vi "ProducerConsumerEvents_Queue.vi"() -> ()   [LabVIEW 2018]
doc: "Use this template to build a producer/consumer design pattern with events to produce queue items. Use this design pattern instead of the User Interface Event Handler pattern for user interfaces when you want to execute code asynchronously in response to an event without slowing the user interface responsiveness."
panel:
  in  "stop 3":bool
  in  "Enqueue Element 3":bool
  in  "stop 2":bool
  in  "Enqueue Element 2":bool
  out "data (can be any type)":string
  in  "Enqueue Element":bool
  in  "stop":bool
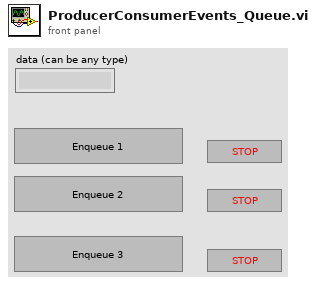
[diagram p1: front panel]
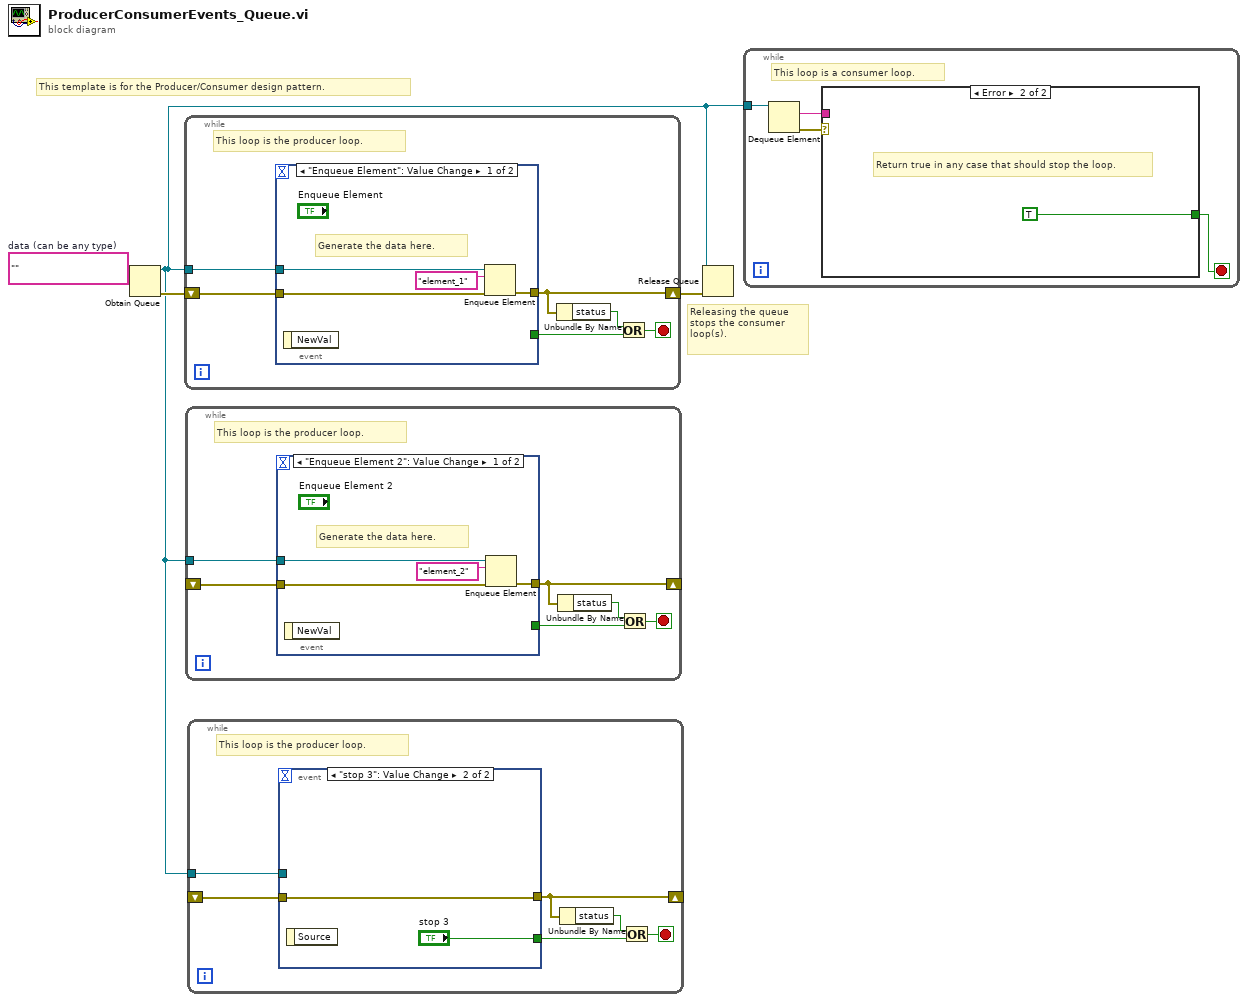
[diagram p0: block diagram]
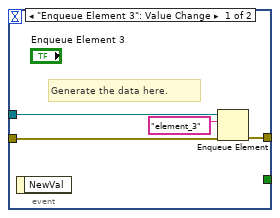
[diagram p2: hidden frame]
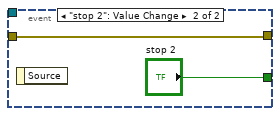
[diagram p3: hidden frame]
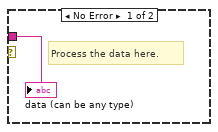
[diagram p4: hidden frame]
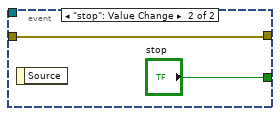
[diagram p5: hidden frame]
diagram:
  w2 = ""  # data (can be any type)
  # "Releasing the queue stops the consumer loop(s)."
  # "This template is for the Producer/Consumer design pattern."
  n1 = Obtain Queue(element data type=w2) -> (queue out=w1:refnum<queue>, error out=w4:errorcluster)  [unwired: 4 in, 1 out]
  n2 = while {
    shift-right: [w6] -> w3
    shift-left: w4 -> [w9]
    tunnel: w1 -> [w10]
    stop <- w7 stop-if-true
    # "This loop is the producer loop."
    n3 = event shown="[0] \"Enqueue Element\": Value Change" {
      selector: _ -> [_ _]
      dyn-events: _ -> [_ _]
      timeout: _ -> [_ _]
      tunnel: w10 -> [w14 _]
      tunnel: w9 -> [w13 w15]
      tunnel: [w12 w15] -> w6
      tunnel: [_ "stop"] -> w8
      event "Enqueue Element": Value Change {
        # "Generate the data here."
        n4 = event-data() -> ()  [unwired: 1 in, 1 out]
        n5 = Enqueue Element(queue=w14, element="element_1", error in (no error)=w13) -> (error out=w12:errorcluster)  [unwired: 1 in, 2 out]
      }
      event "stop": Value Change {
        n6 = event-data() -> ()  [unwired: 1 in, 1 out]
      }
    }
    n7 = Unbundle By Name(w6) -> ("status"=w5:bool)
    n8 = Or(x=w5, y=w8) -> (x .or. y?=w7:bool)
  }
  n9 = while {
    shift-right: [w18] -> _
    shift-left: _ -> [w21]
    tunnel: w1 -> [w22]
    stop <- w19 stop-if-true
    # "This loop is the producer loop."
    n10 = event shown="[0] \"Enqueue Element 2\": Value Change" {
      selector: _ -> [_ _]
      dyn-events: _ -> [_ _]
      timeout: _ -> [_ _]
      tunnel: w22 -> [w26 _]
      tunnel: w21 -> [w25 w27]
      tunnel: [w24 w27] -> w18
      tunnel: [_ "stop 2"] -> w20
      event "Enqueue Element 2": Value Change {
        # "Generate the data here."
        n11 = event-data() -> ()  [unwired: 1 in, 1 out]
        n12 = Enqueue Element(queue=w26, element="element_2", error in (no error)=w25) -> (error out=w24:errorcluster)  [unwired: 1 in, 2 out]
      }
      event "stop 2": Value Change {
        n13 = event-data() -> ()  [unwired: 1 in, 1 out]
      }
    }
    n14 = Unbundle By Name(w18) -> ("status"=w17:bool)
    n15 = Or(x=w17, y=w20) -> (x .or. y?=w19:bool)
  }
  n16 = while {
    shift-right: [w30] -> _
    shift-left: _ -> [w33]
    tunnel: w1 -> [w34]
    stop <- w31 stop-if-true
    # "This loop is the producer loop."
    n17 = event shown="[1] \"stop 3\": Value Change" {
      selector: _ -> [_ _]
      dyn-events: _ -> [_ _]
      timeout: _ -> [_ _]
      tunnel: w34 -> [w38 _]
      tunnel: w33 -> [w37 w39]
      tunnel: [w36 w39] -> w30
      tunnel: [_ "stop 3"] -> w32
      event "Enqueue Element 3": Value Change {
        # "Generate the data here."
        n18 = event-data() -> ()  [unwired: 1 in, 1 out]
        n19 = Enqueue Element(queue=w38, element="element_3", error in (no error)=w37) -> (error out=w36:errorcluster)  [unwired: 1 in, 2 out]
      }
      event "stop 3": Value Change {
        n20 = event-data() -> ()  [unwired: 1 in, 1 out]
      }
    }
    n21 = Unbundle By Name(w30) -> ("status"=w29:bool)
    n22 = Or(x=w29, y=w32) -> (x .or. y?=w31:bool)
  }
  n23 = Release Queue(queue=w1, error in (no error)=w3) -> ()  [unwired: 1 in, 3 out]
  n24 = while {
    tunnel: w1 -> [w44]
    stop <- w41 stop-if-true
    # "This loop is a consumer loop."
    n25 = Dequeue Element(queue=w44) -> (element=w42:string, error out=w43:errorcluster)  [unwired: 2 in, 2 out]
    n26 = case shown="Error" w43 {
      tunnel: w42 -> [w45 _]
      tunnel: [_ TRUE] -> w41
      frame No Error {
        # "Process the data here."
        "data (can be any type)" <- w45
      }
      frame Error {
        # "Return true in any case that should stop the loop."
      }
    }
  }
